vi "Variable BX.vi"() -> ()   [LabVIEW 2020]
panel:
  in  "BX":dbl
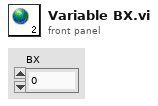
[diagram p1: front panel]
diagram:
